vi "Autonomous Independent.vi"   [LabVIEW 2018]
doc: "This VI is called when autonomous begins, and will automatically be terminated when autonomous ends. You can carry out timed or sensor driven robot movement independently without needing to return to the caller."
uses:
  <vilib>/Rock Robotics/Network Tables/NT Read String Array.vi
  Globals.vi
panel:
  # "Be sure to right-click and choose Data Operations>>Make Current Value default if you want to save the array values with the VI"
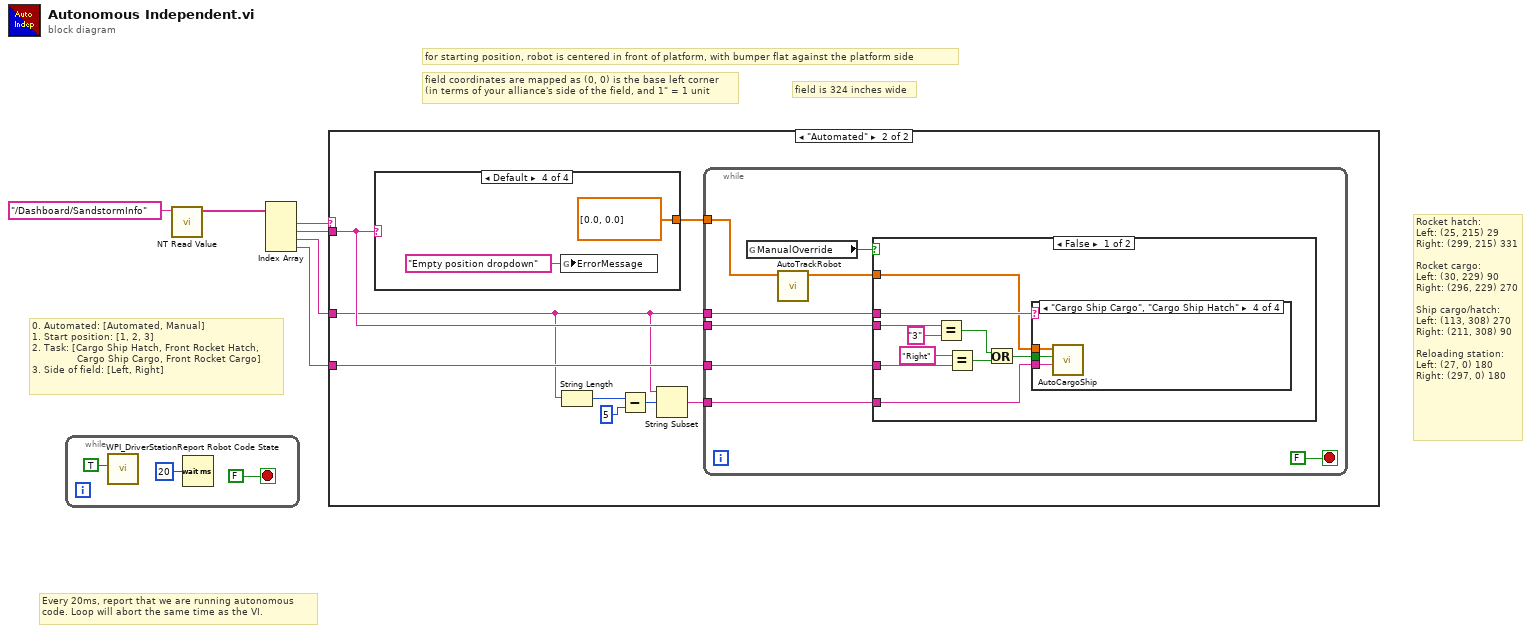
[diagram p0: block diagram]
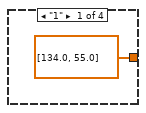
[diagram p3: hidden frame]
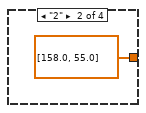
[diagram p4: hidden frame]
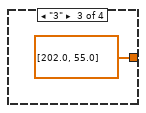
[diagram p5: hidden frame]
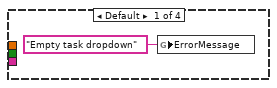
[diagram p6: hidden frame]
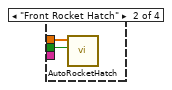
[diagram p7: hidden frame]
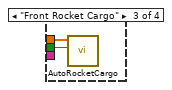
[diagram p8: hidden frame]
diagram:
  # "Rocket hatch:\nLeft: (25, 215) 29\nRight: (299, 215) 331\n\nRocket cargo:\nLeft: (30, 229) 90\nRight: (296, 229) 270\n\nShip cargo/hatch:\nLeft: (113, 308) 270\nRight: (211, 308) 90\n\nReloading station:\nLeft: (27, 0) 180\nRight: (297, 0) 180"
  # "field is 324 inches wide"
  # "for starting position, robot is centered in front of platform, with bumper flat against the platform side"
  # "field coordinates are mapped as (0, 0) is the base left corner\n(in terms of your alliance's side of the field, and 1\" = 1 unit"
  # "0. Automated: [Automated, Manual]\n1. Start position: [1, 2, 3]\n2. Task: [Cargo Ship Hatch, Front Rocket Hatch,\n               Cargo Ship Cargo, Front Rocket Cargo]\n3. Side of field: [Left, Right]"
  # "Every 20ms, report that we are running autonomous\ncode. Loop will abort the same time as the VI."
  n1 = while {
    stop <- FALSE stop-if-true
    n2 = call <vilib>:"WPI_DriverStationReport Robot Code State.vi"("Autonomous"=TRUE) -> ()  [unwired: 10 in, 1 out]
    n3 = Wait (ms)(milliseconds to wait=u32 20) -> ()  [unwired: 1 out]
  }
  n4 = call-poly <vilib>:"NT Read Value.vi"("Name"="/Dashboard/SandstormInfo") -> ("String Array"=w5:string[])  [unwired: 9 in, 1 out]
  n5 = Index Array(array=w5) -> (element #1=w3:string, element #2=w4:string, element #3=w2:string, element #4=w1:string)  [unwired: 4 in]
  n6 = case shown="\"Automated\"" w3 {
    tunnel: w4 -> [_ w16]
    tunnel: w2 -> [_ w10]
    tunnel: w1 -> [_ w15]
    frame "Manual", Default {
    }
    frame "Automated" {
      n7 = case shown="Default" w16 {
        tunnel: [dbl[] [134.0, 55.0] dbl[] [158.0, 55.0] dbl[] [202.0, 55.0] dbl[] [0.0, 0.0]] -> w17
        frame "1" {
        }
        frame "2" {
        }
        frame "3" {
        }
        frame Default {
          n8 = global write "Globals.vi" "ErrorMessage"("Empty position dropdown" ("ErrorMessage")) -> ()
        }
      }
      n9 = String Length(string=w10) -> (length=w13:i32)
      n10 = Subtract(x=w13, y=5) -> (x-y=w14:i32)
      n11 = String Subset(string=w10, offset (0)=w14) -> (substring=w11:string)  [unwired: 1 in]
      n12 = while {
        tunnel: w17 -> [w29]
        tunnel: w10 -> [w28]
        tunnel: w15 -> [w27]
        tunnel: w16 -> [w26]
        tunnel: w11 -> [w23]
        stop <- FALSE stop-if-true
        n13 = global read "Globals.vi" "ManualOverride"() -> (w24:bool)
        n14 = call "AutoTrackRobot.vi"("StartCoordinates"=w29) -> ("Coordinates"=w25:dbl[])  [unwired: 10 in]
        n15 = case shown="False" w24 {
          tunnel: w28 -> [w36 _]
          tunnel: w27 -> [w40 _]
          tunnel: w26 -> [w39 _]
          tunnel: w25 -> [w34 _]
          tunnel: w23 -> [w33 _]
          frame False {
            n16 = Equal?(x=w39, y="3") -> (x = y?=w32:bool)
            n17 = Equal?(x="Right", y=w40) -> (x = y?=w31:bool)
            n18 = Or(x=w32, y=w31) -> (x .or. y?=w35:bool)
            n19 = case shown="\"Cargo Ship Cargo\", \"Cargo Ship Hatch\"" w36 {
              tunnel: w35 -> [_ w42 w45 w47]
              tunnel: w34 -> [_ w43 w44 w48]
              tunnel: w33 -> [_ _ _ w46]
              frame Default {
                n20 = global write "Globals.vi" "ErrorMessage"("Empty task dropdown" ("ErrorMessage")) -> ()
              }
              frame "Front Rocket Hatch" {
                n21 = call "AutoRocketHatch.vi"("RightSideOfField?"=w42, "Coordinates"=w43) -> ()  [unwired: 10 in]
              }
              frame "Front Rocket Cargo" {
                n22 = call "AutoRocketCargo.vi"("RightSideOfField?"=w45, "Coordinates"=w44) -> ()  [unwired: 10 in]
              }
              frame "Cargo Ship Cargo", "Cargo Ship Hatch" {
                n23 = call "AutoCargoShip.vi"("Type"=w46, "RightSideOfField?"=w47, "Coordinates"=w48) -> ()  [unwired: 9 in]
              }
            }
          }
          frame True {
          }
        }
      }
    }
  }
